vi "HistoricodePartidas.vi"() -> ()   [LabVIEW 2011]
doc: "VI que mostra o histórico de partidas, ou seja, nome dos jogadores, as jogadas de cada um e quem venceu ou se houve empate."
uses:
  <vilib>/Utility/sysdir.llb/System Directory Type.ctl
panel:
  in  "LimparHistorico":bool
  in  "OK":bool
  out "Histórico":string
  # "Histórico de Partidas"
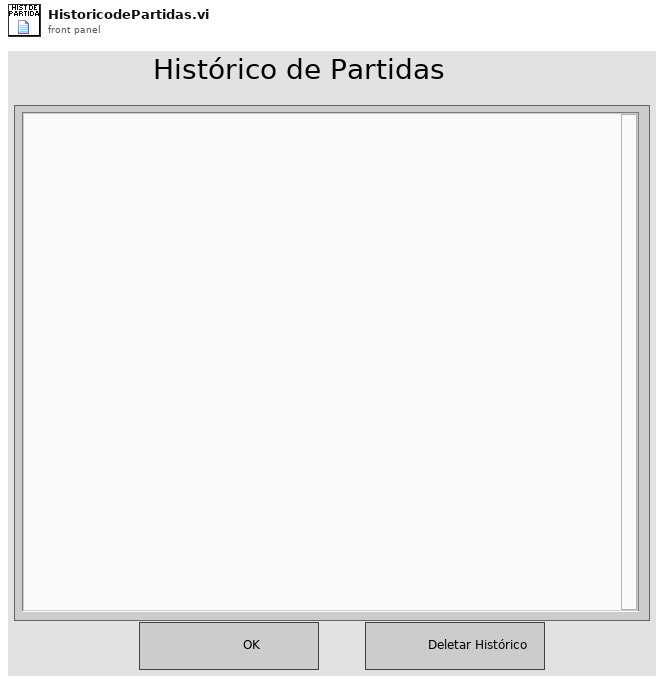
[diagram p1: front panel]
types:
  T1 = enum16{"open", "replace", "create", "open or create", "replace or create", "replace or create with confirmation"}
  T2 = typedef "System Directory Type.ctl" = i32
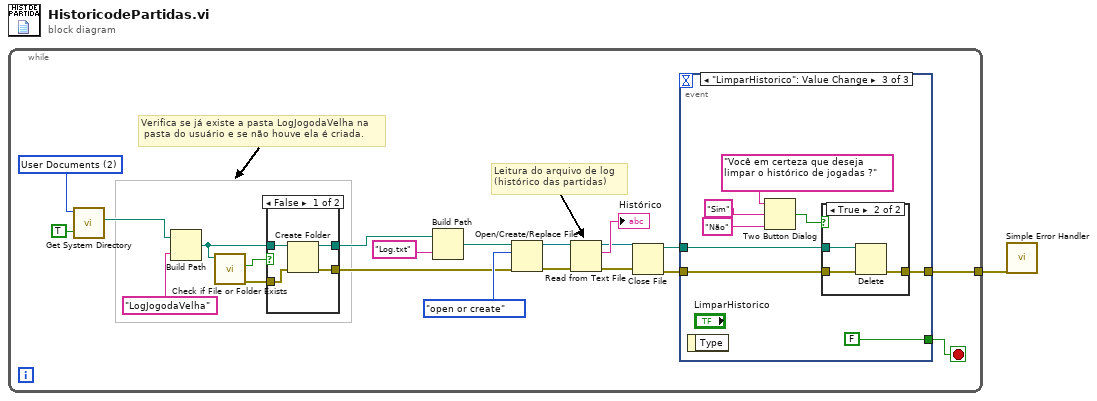
[diagram p0: block diagram]
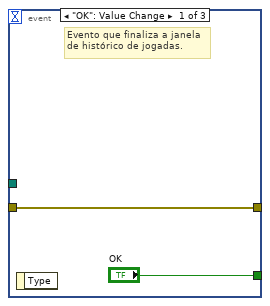
[diagram p3: hidden frame]
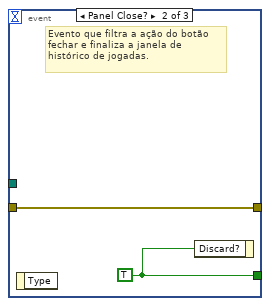
[diagram p4: hidden frame]
diagram:
  n1 = while {
    tunnel: [w14] -> w1
    stop <- w21 stop-if-true
    w13 = T2 2 items=["User Home"=0, "User Desktop"=1, "User Documents"=2, "User Application Data"=3, "User Preferences"=4, "User Temporary"=5, "Public Documents"=6, "Public Application Data"=7, "Public Preferences"=8, "Public Cache"=13, "System Core Libraries"=9, "System Installed Libraries"=10, "Application Files"=11, "Boot Volume Root"=12] ("system directory type")
    # "Leitura do arquivo de log\n(histórico das partidas)"
    # "Verifica se já existe a pasta LogJogodaVelha na\n pasta do usuário e se não houve ela é criada."
    n2 = call <vilib>:"Get System Directory.vi"("create directory if not found? (F)"=TRUE, "system directory type"=w13) -> ("system directory"=w11:path)  [unwired: 9 in]
    n3 = Build Path(base path=w11, name or relative path="LogJogodaVelha") -> (appended path=w9:path)
    n4 = call <vilib>:"Check if File or Folder Exists.vi"("path"=w9) -> ("error out"=w8:errorcluster, "file or folder exists?"=w7:bool)  [unwired: 8 in, 1 out]
    n5 = case shown="False" w7 {
      tunnel: [w26 w28] -> w4
      tunnel: [w25 w27] -> w6
      tunnel: w9 -> [w24 w28]
      tunnel: w8 -> [w23 w27]
      frame False {
        n6 = Create Folder(path (use dialog)=w24, error in=w23) -> (created path=w26:path, error out=w25:errorcluster)  [unwired: 1 in, 1 out]
      }
      frame True {
      }
    }
    n7 = Build Path(base path=w4, name or relative path="Log.txt") -> (appended path=w3:path)
    n8 = Open/Create/Replace File(file path (use dialog)=w3, error in=w6, operation (0:open)=T1."open or create") -> (refnum out=w19:refnum<file>, error out=w18:errorcluster)  [unwired: 3 in, 1 out]
    n9 = Read from Text File(file (use dialog)=w19, error in=w18) -> (refnum out=w17:refnum<file>, text=→"Histórico":string, error out=w16:errorcluster)  [unwired: 2 in, 1 out]
    n10 = Close File(refnum=w17, error in=w16) -> (path=w2:path, error out=w15:errorcluster)
    n11 = event shown="[2] \"LimparHistorico\": Value Change" {
      selector: _ -> [_ _ _]
      dyn-events: _ -> [_ _ _]
      timeout: _ -> [_ _ _]
      tunnel: ["OK" w31 FALSE ("Discard?")] -> w21
      tunnel: w15 -> [w29 w32 w39]
      tunnel: [w29 w32 w38] -> w14
      tunnel: w2 -> [_ _ w33]
      event "OK": Value Change {
        # "Evento que finaliza a janela\nde histórico de jogadas."
        n12 = event-data() -> ()  [unwired: 1 in, 1 out]
      }
      event Panel Close? {
        w31 = TRUE ("Discard?")
        # "Evento que filtra a ação do botão \nfechar e finaliza a janela de\nhistórico de jogadas."
        n13 = event-data() -> ()  [unwired: 1 in, 1 out]
        n14 = event-data("Discard?"=w31) -> ()  [unwired: 1 in, 1 out]
      }
      event "LimparHistorico": Value Change {
        n15 = event-data() -> ()  [unwired: 1 in, 1 out]
        n16 = Two Button Dialog(message="Você em certeza que deseja limpar o histórico de jogadas ?", 1:"Não" ("F button name (\"Cancel\")"), 2:"Sim" ("T button name (\"OK\")")) -> (T button?=w37:bool)
        n17 = case shown="True" w37 {
          tunnel: w39 -> [w41 w44]
          tunnel: [w41 w43] -> w38
          tunnel: w33 -> [_ w42]
          frame False {
          }
          frame True {
            n18 = Delete(path (use dialog)=w42, error in=w44) -> (error out=w43:errorcluster)  [unwired: 3 in, 2 out]
          }
        }
      }
    }
  }
  n19 = call <vilib>:"Simple Error Handler.vi"("error in (no error)"=w1) -> ()  [unwired: 4 in, 5 out]
